vi "Main_UI.vi"() -> ()   [LabVIEW 2009]
uses:
  UI Control/UI State.ctl
  UI Control/LCOD_FP Command.ctl
  Global/Global 1.vi
panel:
  in  "Full Test?":bool=TRUE
  out "Software Title":string
  in  "Stop":bool
  in  "Clear":bool
  out "YIELD (%)":dbl format="%_3g"
  out "TOTAL":dbl
  out "FAILED":dbl
  out "PASS":dbl
  in  "Reset":bool
  in  "Mode":bool=TRUE
  in  "Setting":bool
  in  "Test":bool
  in  "Exit":bool
  out "Message":string="Idle: Train Mode"
  out "Status":bool caption="״̬"
  out "Time":string="1:17:42 PM"
  out "Date":string="Sunday, September 28, 2008"
  # "Production"
  # "Maintenance"
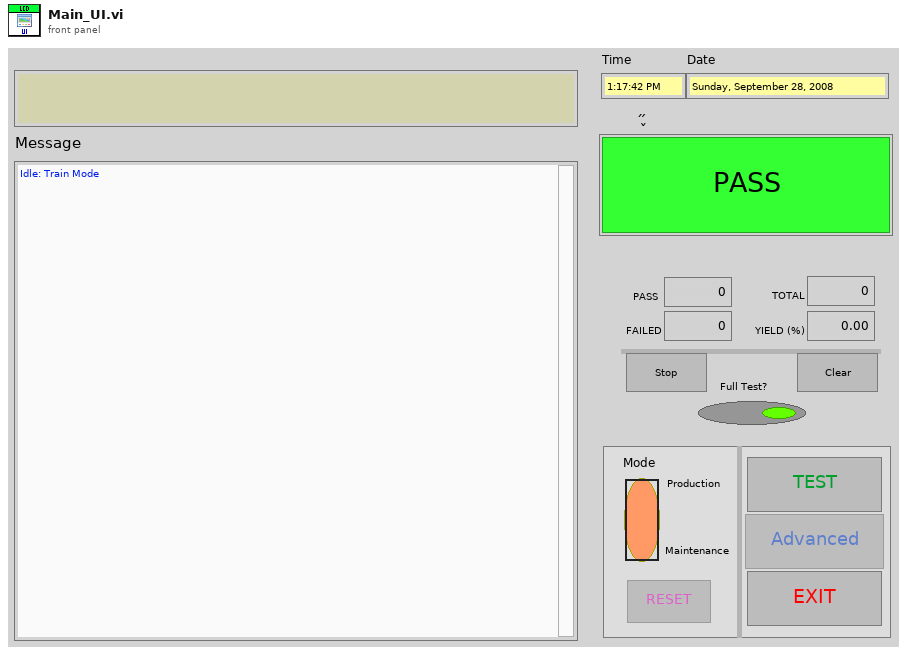
[diagram p1: front panel]
types:
  T1 = typedef "UI State.ctl" = enum16{"Initialization", "Run", "Post Condition"}
  T2 = typedef "LCOD_FP Command.ctl" = enum16{"Under Range", "Get FP Setting", "HadError", "ResetPressed", "DisplayMsg", "StartPressed", "SetGood", "SetNoGood", "SetIntesting", "Over Range"}
  T3 = typedef "LCOD_Stack Queue GUI Command.ctl" = enum16{"No Change", "HadError", "ResetPressed", "DisplayMsg", "StartPressed", "SetGood", "SetNoGood", "SetIntesting"}
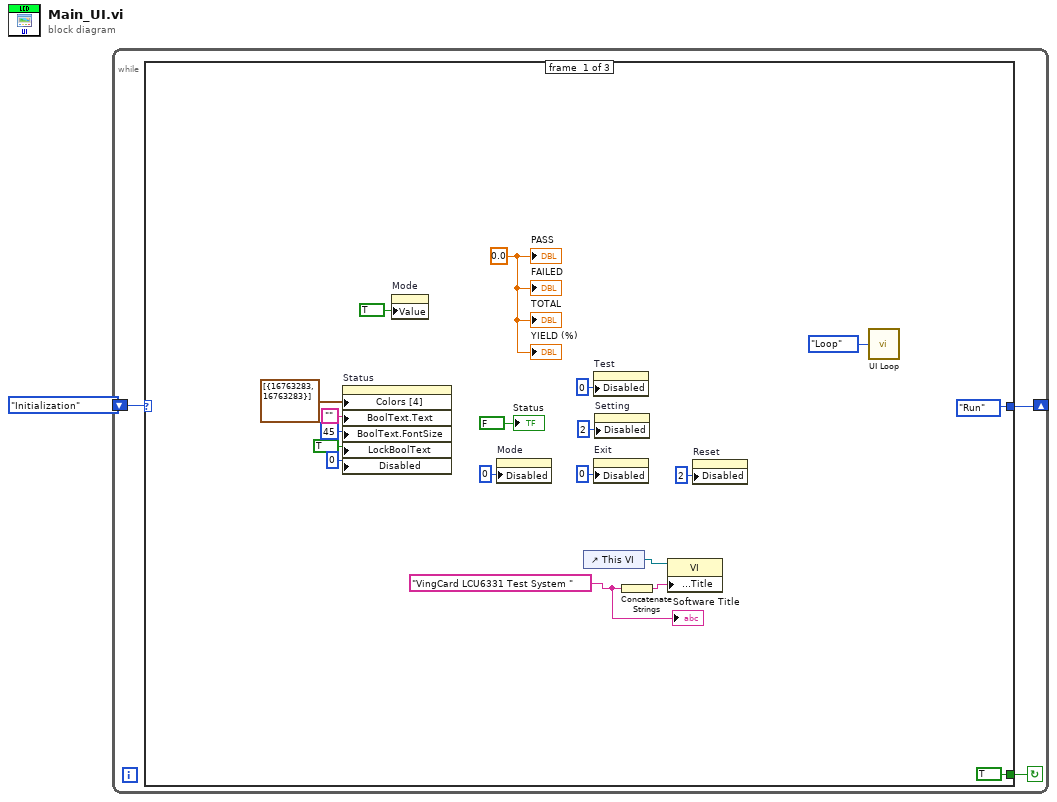
[diagram p0: block diagram]
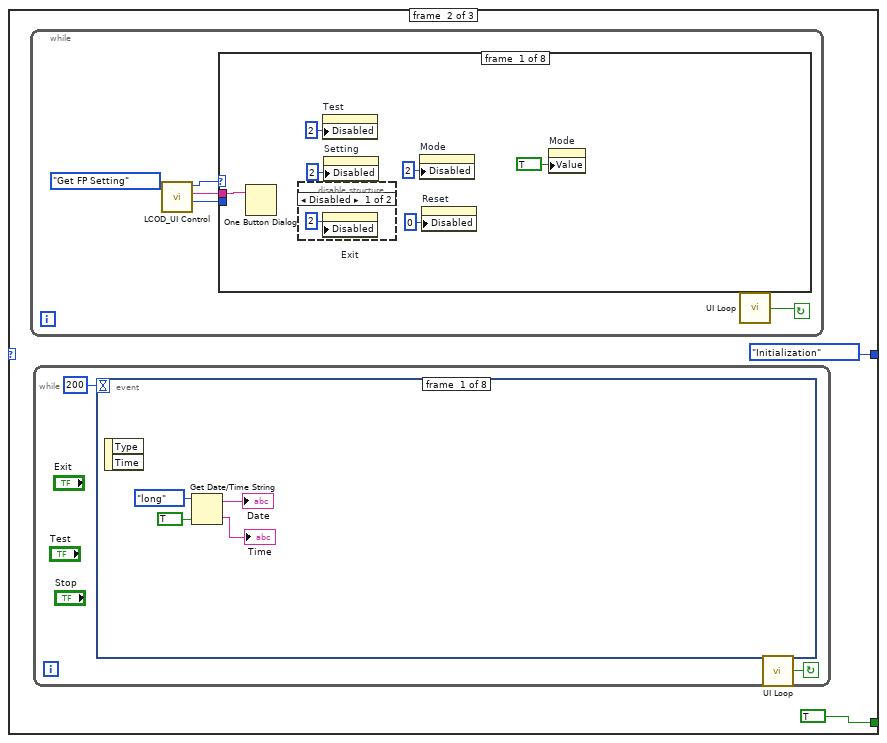
[diagram p2: hidden frame]
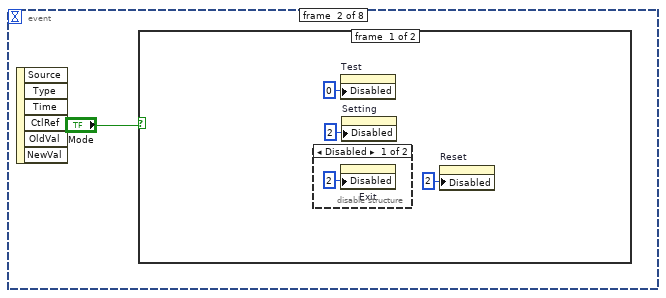
[diagram p3: hidden frame]
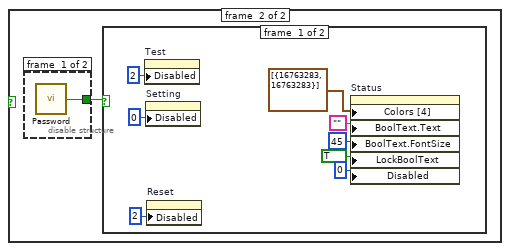
[diagram p5: hidden frame]
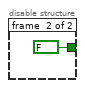
[diagram p6: hidden frame]
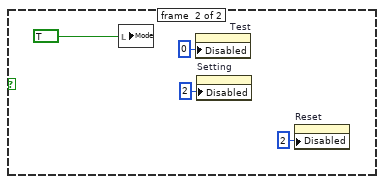
[diagram p7: hidden frame]
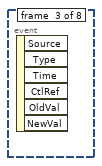
[diagram p8: hidden frame]
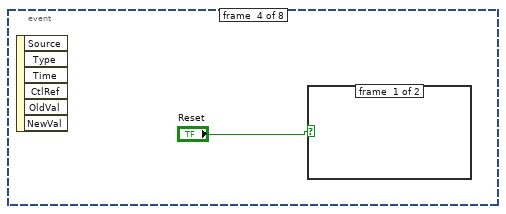
[diagram p9: hidden frame]
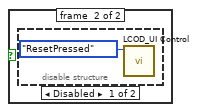
[diagram p10: hidden frame]
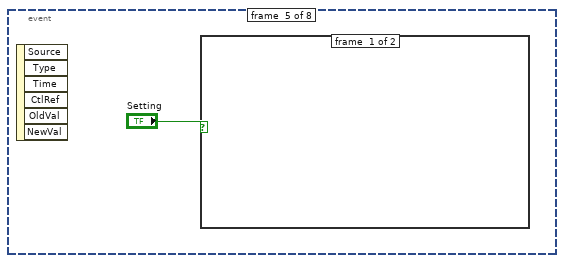
[diagram p12: hidden frame]
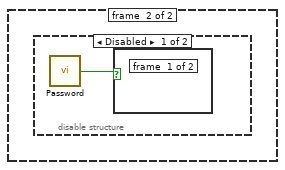
[diagram p13: hidden frame]
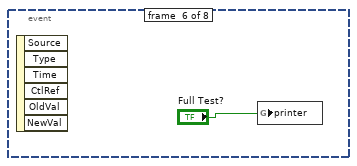
[diagram p16: hidden frame]
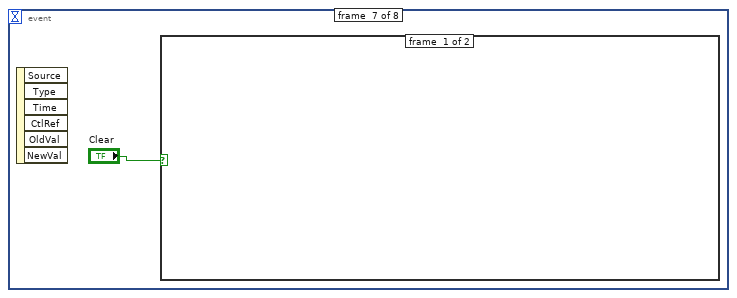
[diagram p17: hidden frame]
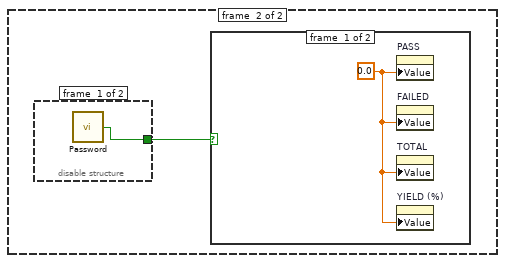
[diagram p18: hidden frame]
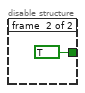
[diagram p19: hidden frame]
diagram:
  n1 = while {
    shift-right: [w3] -> _
    shift-left: UI_State."Initialization" ("UI State") -> [w4]
    stop <- w2 continue-if-true
    n2 = case shown="\"Run\"" w4 {
      tunnel: [UI_State."Run" ("UI State") UI_State."Initialization" ("UI State") UI_State."Post Condition" ("UI State")] -> w3
      tunnel: [TRUE TRUE FALSE] -> w2
      frame #0 {
        w5 = "VingCard LCU6331 Test System " ("string")
        w21 = 0.0 ("YIELD (%)")
        n3 = property on="Status" class="Bool (strict)"("Colors [4]"=cluster{u32, u32}[] [{16763283, 16763283}], "BoolText.Text"="", "BoolText.FontSize"=u32 45 ("Boolean Text.Font:Size"), "LockBoolText"=TRUE ("Lock Boolean Text In Center"), "Disabled"=u8 0) -> ()  [unwired: 2 in, 2 out]
        n4 = property on="Mode" class="Bool (strict)"("Value"=TRUE ("Mode")) -> ()  [unwired: 2 in, 2 out]
        n5 = property on="Mode" class="Bool (strict)"("Disabled"=u8 0) -> ()  [unwired: 2 in, 2 out]
        n6 = control-ref of="This VI"() -> (w7:refnum<vi>)
        n7 = property on="Test" class="Bool"("Disabled"=u8 0) -> ()  [unwired: 2 in, 2 out]
        n8 = property on="Exit" class="Bool"("Disabled"=u8 0) -> ()  [unwired: 2 in, 2 out]
        n9 = property on="Setting" class="Bool"("Disabled"=u8 2) -> ()  [unwired: 2 in, 2 out]
        n10 = Concatenate Strings(w5) -> (w8:string)
        n11 = property class="VI"(reference=w7, "Front Panel.Title"=w8) -> ()  [unwired: 1 in, 2 out]
        n12 = property on="Reset" class="Bool"("Disabled"=u8 2) -> ()  [unwired: 2 in, 2 out]
        n13 = call "UI Loop.vi"("Loop"=enum16{"Do Nothing", "Loop", "Stop"}."Loop") -> ()  [unwired: 5 out]
        "YIELD (%)" <- w21
        "FAILED" <- w21
        "TOTAL" <- w21
        "PASS" <- w21
        "Status" <- FALSE ("Test Result")
        "Software Title" <- w5
      }
      frame #1 {
        n14 = while {
          stop <- w69 continue-if-true
          n15 = call "LCOD_UI Control.vi"("Command"=LCOD_FP_Command."Get FP Setting") -> ("Numeric Out"=w70:i32, "String Out"=w71:string, "GUI Command Out"=w72:T3)  [unwired: 2 in, 3 out]
          n16 = case shown="\"DisplayMsg\"" w72 {
            tunnel: w71 -> [w74 _ w87 _ _ _ w131 _]
            tunnel: w70 -> [_ _ _ _ _ _ _ _]
            frame #0 {
              n17 = One Button Dialog(message=w74) -> ()  [unwired: 2 out]
              n18 = disable-structure shown="Disabled" {
                frame #0 {
                  n19 = property on="Exit" class="Bool"("Disabled"=u8 2) -> ()  [unwired: 2 in, 2 out]
                }
                frame #1 {
                }
              }
              n20 = property on="Test" class="Bool"("Disabled"=u8 2) -> ()  [unwired: 2 in, 2 out]
              n21 = property on="Setting" class="Bool"("Disabled"=u8 2) -> ()  [unwired: 2 in, 2 out]
              n22 = property on="Mode" class="Bool (strict)"("Disabled"=u8 2) -> ()  [unwired: 2 in, 2 out]
              n23 = property on="Reset" class="Bool"("Disabled"=u8 0) -> ()  [unwired: 2 in, 2 out]
              n24 = property on="Mode" class="Bool (strict)"("Value"=TRUE ("Mode")) -> ()  [unwired: 2 in, 2 out]
            }
            frame #1 {
              n25 = property on="Mode" class="Bool (strict)"("Disabled"=u8 0) -> ()  [unwired: 2 in, 2 out]
              n26 = property on="Test" class="Bool"("Disabled"=u8 0) -> ()  [unwired: 2 in, 2 out]
              n27 = property on="Setting" class="Bool"("Disabled"=u8 2) -> ()  [unwired: 2 in, 2 out]
              n28 = property on="Reset" class="Bool"("Disabled"=u8 2) -> ()  [unwired: 2 in, 2 out]
              n29 = property on="Mode" class="Bool (strict)"("Value"=TRUE ("Mode")) -> ()  [unwired: 2 in, 2 out]
            }
            frame #2 {
              n30 = case shown="True" TRUE {
                tunnel: [w89 w95] -> w88
                tunnel: w87 -> [w89 w94]
                frame #0 {
                }
                frame #1 {
                  n31 = property on="Message" class="Str"() -> ("Text.Scroll Position"=w92:u32)  [unwired: 2 in, 2 out]
                  n32 = property on="Message" class="Str"() -> ("Value"=w93:string)  [unwired: 2 in, 2 out]
                  n33 = String Length(string=w93) -> (length=w96:i32)
                  n34 = Subtract(x=w96, y=500) -> (x-y=w98:i32)
                  n35 = Add(x=w92, y=u32 250) -> (x+y=w90:u32)
                  n36 = Max & Min(x=w98, y=0) -> (max(x,y)=w100:i32)  [unwired: 1 out]
                  n37 = property on="Message" class="Str"("Text.Scroll Position"=w90) -> ()  [unwired: 2 in, 2 out]
                  n38 = String Subset(string=w93, offset (0)=w100) -> (substring=w101:string)  [unwired: 1 out]
                  n39 = Concatenate Strings(w101, "\r\n", w94) -> (w95:string)
                }
              }
              "Message" <- w88
            }
            frame #3 {
              n40 = property on="Message" class="Str"("Value"="Start pressed\n" ("Message")) -> ()  [unwired: 2 in, 2 out]
            }
            frame #4 {
              n41 = property on="PASS" class="DigNum (strict)"() -> ("Value"=w112:dbl)  [unwired: 2 in, 2 out]
              n42 = property on="TOTAL" class="DigNum (strict)"() -> ("Value"=w111:dbl)  [unwired: 2 in, 2 out]
              n43 = Increment(x=w112) -> (x+1=w110:dbl)
              n44 = Increment(x=w111) -> (x+1=w109:dbl)
              n45 = Divide(x=w110, y=w109) -> (x/y=w107:dbl)
              n46 = property on="PASS" class="DigNum (strict)"("Value"=w110) -> ()  [unwired: 2 in, 2 out]
              n47 = property on="TOTAL" class="DigNum (strict)"("Value"=w109) -> ()  [unwired: 2 in, 2 out]
              n48 = Multiply(x=w107, y=100.0) -> (x*y=w106:dbl)
              n49 = property on="YIELD (%)" class="DigNum (strict)"("Value"=w106) -> ()  [unwired: 2 in, 2 out]
              n50 = property on="Status" class="Bool (strict)"("Colors [4]"=cluster{u32, u32}[] [{3407667, 3407667}], "BoolText.Text"="PASS" ("String Out"), "BoolText.FontSize"=u32 45 ("Boolean Text.Font:Size"), "LockBoolText"=TRUE ("Lock Boolean Text In Center"), "Disabled"=u8 0, "Blinking"=FALSE) -> ()  [unwired: 2 in, 2 out]
            }
            frame #5 {
              n51 = property on="TOTAL" class="DigNum (strict)"() -> ("Value"=w125:dbl)  [unwired: 2 in, 2 out]
              n52 = property on="FAILED" class="DigNum (strict)"() -> ("Value"=w126:dbl)  [unwired: 2 in, 2 out]
              n53 = property on="PASS" class="DigNum (strict)"() -> ("Value"=w119:dbl)  [unwired: 2 in, 2 out]
              n54 = Increment(x=w125) -> (x+1=w123:dbl)
              n55 = Increment(x=w126) -> (x+1=w124:dbl)
              n56 = Divide(x=w119, y=w123) -> (x/y=w121:dbl)
              n57 = property on="FAILED" class="DigNum (strict)"("Value"=w124) -> ()  [unwired: 2 in, 2 out]
              n58 = property on="TOTAL" class="DigNum (strict)"("Value"=w123) -> ()  [unwired: 2 in, 2 out]
              n59 = Multiply(x=w121, y=100.0) -> (x*y=w120:dbl)
              n60 = property on="YIELD (%)" class="DigNum (strict)"("Value"=w120) -> ()  [unwired: 2 in, 2 out]
              n61 = property on="Status" class="Bool (strict)"("Colors [4]"=cluster{u32, u32}[] [{16711680, 16711680}], "BoolText.Text"="Failed" ("Boolean Text.Text"), "BoolText.FontSize"=u32 45 ("Boolean Text.Font:Size"), "LockBoolText"=TRUE ("Lock Boolean Text In Center"), "Disabled"=u8 0, "Blinking"=FALSE) -> ()  [unwired: 2 in, 2 out]
            }
            frame #6 {
              n62 = property on="Status" class="Bool (strict)"("Colors [4]"=cluster{u32, u32}[] [{3394560, 1244}], "BoolText.Text"=w131, "BoolText.FontSize"=u32 22 ("Boolean Text.Font:Size"), "LockBoolText"=TRUE ("Lock Boolean Text In Center"), "Disabled"=u8 0, "Blinking"=TRUE) -> ()  [unwired: 2 in, 2 out]
            }
            frame #7 {
            }
          }
          n63 = call "UI Loop.vi"() -> ("Loop Out"=w69:bool)  [unwired: 1 in, 4 out]
        }
        n64 = while {
          stop <- w26 continue-if-true
          n65 = event shown="[5] \"Full Test?\": Value Change" {
            selector: _ -> [_ _ _ _ _ _ _ _]
            dyn-events: _ -> [_ _ _ _ _ _ _ _]
            timeout: 200 -> [_ _ _ _ _ _ _ _]
            event #0 {
              n66 = event-data() -> ()  [unwired: 3 out]
              n67 = Get Date/Time String(date format (0)=enum16{"short", "long", "abbreviated"}."long", want seconds? (F)=TRUE) -> (date string=→"Date":string, time string=→"Time":string)  [unwired: 1 out]
            }
            event #1 {
              n68 = event-data() -> ()  [unwired: 7 out]
              n69 = case shown="False" "Mode" {
                frame #0 {
                  n70 = disable-structure shown="Disabled" {
                    frame #0 {
                      n71 = property on="Exit" class="Bool"("Disabled"=u8 2) -> ()  [unwired: 2 in, 2 out]
                    }
                    frame #1 {
                    }
                  }
                  n72 = property on="Test" class="Bool"("Disabled"=u8 0) -> ()  [unwired: 2 in, 2 out]
                  n73 = property on="Setting" class="Bool"("Disabled"=u8 2) -> ()  [unwired: 2 in, 2 out]
                  n74 = property on="Reset" class="Bool"("Disabled"=u8 2) -> ()  [unwired: 2 in, 2 out]
                }
                frame #1 {
                  n75 = disable-structure shown="Enabled" {
                    disable-tunnel: [w38 FALSE ("Cancel")] -> w37
                    frame #0 {
                      n76 = call "Password.vi"() -> ("Cancel"=w38:bool)  [unwired: 3 out]
                    }
                    frame #1 {
                    }
                  }
                  n77 = case shown="False" w37 {
                    frame #0 {
                      n78 = property on="Test" class="Bool"("Disabled"=u8 2) -> ()  [unwired: 2 in, 2 out]
                      n79 = property on="Setting" class="Bool"("Disabled"=u8 0) -> ()  [unwired: 2 in, 2 out]
                      n80 = property on="Reset" class="Bool"("Disabled"=u8 2) -> ()  [unwired: 2 in, 2 out]
                      n81 = property on="Status" class="Bool (strict)"("Colors [4]"=cluster{u32, u32}[] [{16763283, 16763283}], "BoolText.Text"="", "BoolText.FontSize"=u32 45 ("Boolean Text.Font:Size"), "LockBoolText"=TRUE ("Lock Boolean Text In Center"), "Disabled"=u8 0) -> ()  [unwired: 2 in, 2 out]
                    }
                    frame #1 {
                      n82 = local write "Mode"(TRUE ("Mode")) -> ()
                      n83 = property on="Test" class="Bool"("Disabled"=u8 0) -> ()  [unwired: 2 in, 2 out]
                      n84 = property on="Setting" class="Bool"("Disabled"=u8 2) -> ()  [unwired: 2 in, 2 out]
                      n85 = property on="Reset" class="Bool"("Disabled"=u8 2) -> ()  [unwired: 2 in, 2 out]
                    }
                  }
                }
              }
            }
            event #2 {
              n86 = event-data() -> ()  [unwired: 7 out]
            }
            event #3 {
              n87 = event-data() -> ()  [unwired: 7 out]
              n88 = case shown="True" "Reset" {
                frame #0 {
                }
                frame #1 {
                  n89 = disable-structure shown="Disabled" {
                    frame #0 {
                      n90 = call "LCOD_UI Control.vi"("Command"=LCOD_FP_Command."ResetPressed") -> ()  [unwired: 2 in, 6 out]
                    }
                    frame #1 {
                    }
                  }
                }
              }
            }
            event #4 {
              n91 = event-data() -> ()  [unwired: 7 out]
              n92 = case shown="True" "Setting" {
                frame #0 {
                }
                frame #1 {
                  n93 = disable-structure shown="Disabled" {
                    frame #0 {
                      n94 = call "Password.vi"() -> ("Cancel"=w55:bool)  [unwired: 3 out]
                      n95 = case shown="False" w55 {
                        frame #0 {
                        }
                        frame #1 {
                        }
                      }
                    }
                    frame #1 {
                    }
                  }
                }
              }
            }
            event #5 {
              n96 = event-data() -> ()  [unwired: 7 out]
              n97 = global write "Global 1.vi" "printer"("Full Test?") -> ()
            }
            event #6 {
              n98 = event-data() -> ()  [unwired: 7 out]
              n99 = case shown="True" "Clear" {
                frame #0 {
                }
                frame #1 {
                  n100 = disable-structure shown="Enabled" {
                    disable-tunnel: [w59 TRUE ("Cancel")] -> w58
                    frame #0 {
                      n101 = call "Password.vi"() -> ("Cancel"=w59:bool)  [unwired: 3 out]
                    }
                    frame #1 {
                    }
                  }
                  n102 = case shown="False" w58 {
                    frame #0 {
                      w61 = 0.0 ("PASS")
                      n103 = property on="PASS" class="DigNum (strict)"("Value"=w61) -> ()  [unwired: 2 in, 2 out]
                      n104 = property on="FAILED" class="DigNum (strict)"("Value"=w61) -> ()  [unwired: 2 in, 2 out]
                      n105 = property on="TOTAL" class="DigNum (strict)"("Value"=w61) -> ()  [unwired: 2 in, 2 out]
                      n106 = property on="YIELD (%)" class="DigNum (strict)"("Value"=w61) -> ()  [unwired: 2 in, 2 out]
                    }
                    frame #1 {
                    }
                  }
                }
              }
            }
            event #7 {
              n107 = event-data() -> ()  [unwired: 4 out]
              n108 = while {
                tunnel: enum16{"Do Nothing", "Loop", "Stop"}."Stop" ("Loop") -> [w66]
                tunnel: [w66] -> w62
                stop <- w68 continue-if-true
                n109 = call "Main Control Loop.vi"("Loop"=w66) -> ("Loop Out"=w68:bool)  [unwired: 4 out]
                n110 = Wait Until Next ms Multiple(millisecond multiple=u32 100) -> ()  [unwired: 1 out]
              }
              n111 = call "LCOD_UI Control.vi"("String In"="Software is closing....", "Command"=LCOD_FP_Command."DisplayMsg") -> ()  [unwired: 1 in, 6 out]
              n112 = call "UI Loop.vi"("Loop"=w62) -> ()  [unwired: 5 out]
            }
          }
          n113 = call "UI Loop.vi"() -> ("Loop Out"=w26:bool)  [unwired: 1 in, 4 out]
        }
      }
      frame #2 {
      }
    }
  }
